vi "HumanExecute.vi"(8 "error in (no error)":errorcluster) -> (0 "error out":errorcluster)   [LabVIEW 2023]
doc: "Execute for Human\n\ninput:\n error in (cluster)\n\noutput:\n error out (cluster)"
uses:
  <vilib>/Rock Robotics/WPI/Joystick/XBox Buttons Indexer.ctl
  <vilib>/Rock Robotics/WPI/ThirdParty/JAS_Junk/TrajLib/VI/BoolCmd_Send_Internal.vi
  <vilib>/Rock Robotics/WPI/ThirdParty/JAS_Junk/TrajLib/VI/BoolCmd_ObtainQueue.vi
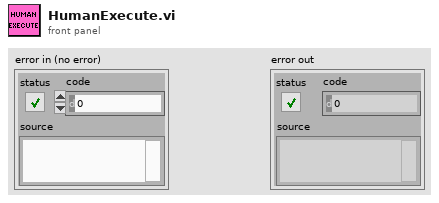
[diagram p1: front panel]
types:
  T1 = typedef "XBox Buttons Indexer.ctl" = enum16{"A", "B", "X", "Y", "Left Bumper", "Right Bumper", "Back", "Start", "Left Joystick", "Right Joystick"}
  T2 = typedef "WPI_JoystickDevRef.ctl" = cluster{"Device":T3}
  T3 = typedef "WPI_JoystickDeviceEnum.ctl" = enum16{"USB 0", "USB 1", "USB 2", "USB 3", "USB 4", "USB 5"}
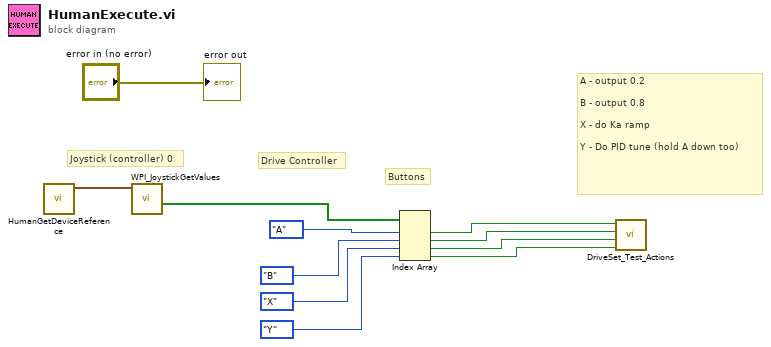
[diagram p0: block diagram]
diagram:
  # "A - output 0.2\n\nB - output 0.8\n\nX - do Ka ramp\n\nY - Do PID tune (hold A down too)"
  # "Buttons"
  # "Joystick (controller) 0"
  # "Drive Controller"
  n1 = call "HumanGetDeviceReference.vi"() -> ("Driver Joy"=w10:T2)  [unwired: 9 in, 2 out]
  n2 = call <vilib>:"WPI_JoystickGetValues.vi"("JoystickDevRef"=w10) -> ("Buttons"=w9:bool[])  [unwired: 6 in, 4 out]
  n3 = Index Array(array=w9, index #1=XBox_Buttons_Indexer."A" ("Nothing"), index #2=XBox_Buttons_Indexer."B" ("Nothing"), index #3=XBox_Buttons_Indexer."X" ("Nothing"), index #4=XBox_Buttons_Indexer."Y" ("Nothing")) -> (element #1=w4:bool, element #2=w3:bool, element #3=w2:bool, element #4=w1:bool)
  n4 = call "DriveSet_Test_Actions.vi"("Do PID test"=w1, "Do Ka  Test"=w2, "Do 0.8 output"=w3, "Do 0.2 output"=w4) -> ()  [unwired: 8 in]
  "error out" <- "error in (no error)"
